vi "Pre_Loop_Initialization_FGV.vi"(8 "error in (no error)":errorcluster, 11 "VI in":refnum<vi>) -> (0 "error out":errorcluster, 3 "User Event out":refnum<user-event>)   [LabVIEW 2024, in "MANUAL_MODE.lvlib"]
doc: "This VI\n------------------------------------------------\nPer_Loop_Initialize\n------------------------------------------------\n-Generate the Communication Queue Reference with FGV.\n-Get the Common User Events Reference at Application Level."
uses:
  MANUAL_MODE.lvlib
  PrivateControls/FGV_Queue_Control.ctl
  support/Message Queue/Message Cluster.ctl
  support/Message Queue/Manual Message Queue.lvlib
  UserEvents/Controls/User_Events_Action_Control.ctl
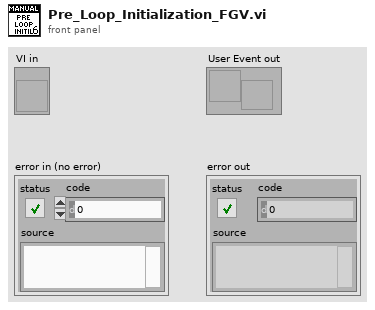
[diagram p1: front panel]
types:
  T1 = typedef "MANUAL_MODE.lvlib/User_Events_Action_Control.ctl" = enum16{"Get", "Create", "Destroy"}
  T2 = typedef "MANUAL_MODE.lvlib/Manual Message Queue.lvlib/Message Cluster.ctl" = cluster{"Message":string, "Message Data":variant}
  T3 = typedef "MANUAL_MODE.lvlib/FGV_Queue_Control.ctl" = enum16{"Release", "Get", "Set"}
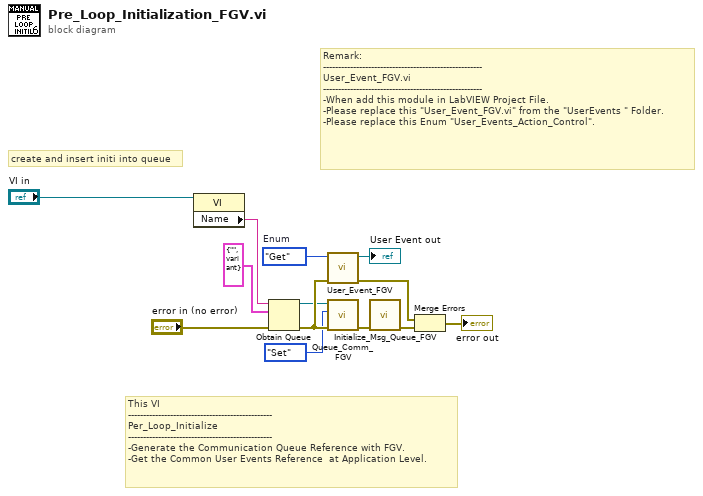
[diagram p0: block diagram]
diagram:
  w8 = User_Events_Action_Control."Get"  # Enum
  # "Remark:\n-----------------------------------------------------\nUser_Event_FGV.vi\n-----------------------------------------------------\n-When add this module in LabVIEW Project File.\n-Please replace this \"User_Event_FGV.vi\" from the \"UserEvents \" Folder.\n-Please replace this Enum \"User_Events_Action_Control\"."
  # "This VI\n------------------------------------------------\nPer_Loop_Initialize\n------------------------------------------------\n-Generate the Communication Queue Reference with FGV.\n-Get the Common User Events Reference  at Application Level."
  # "create and insert initi into queue"
  n1 = property class="VI"(reference="VI in") -> ("Name"=w2:string)  [unwired: 1 in, 2 out]
  n2 = Obtain Queue(name (unnamed)=w2, element data type=T2 {"Message"="", "Message Data"=variant} ("Message Cluster"), error in (no error)="error in (no error)") -> (queue out=w7:refnum<queue>, error out=w9:errorcluster)  [unwired: 2 in, 1 out]
  n3 = call "User_Event_FGV.vi"("error in (no error)"=w9, "Enum"=w8) -> ("error out"=w11:errorcluster, "User Event out"=→"User Event out":refnum<user-event>)  [unwired: 8 in]
  n4 = call "Queue_Comm_FGV.vi"("error in (no error)"=w9, "Enum"=FGV_Queue_Control."Set", "queue in"=w7) -> ("error Out"=w5:errorcluster)  [unwired: 7 in, 1 out]
  n5 = call "Initialize_Msg_Queue_FGV.vi"("error in (no error)"=w5) -> ("error out"=w12:errorcluster)  [unwired: 10 in]
  n6 = Merge Errors(w11, w12) -> (→"error out":errorcluster)
